vi "Spanning.vi"(6 "Numeric":i32, 8 "error in":errorcluster, 9 "TDMS File Ref":path, 10 "Log Start Time":timestamp, 11 "File Log Specification":T1={"Directory"=path "", "Groups"=[], "Buffer Size"=0, "Properties"=[], "Pretrigger"=FALSE, "Name"="", "Timestamp"=FALSE, "Error"=0, "Auto Open"=FALSE, "File Node Ref"=18446744073709551615, "Archive"=FALSE, "Archive Directory"=path "", "Span by Time"=FALSE, "Maximum Log Time"=86400, "Span by Size"=FALSE, "Maximum File Size"=100000} {"File Node Ref" format="%.0x"}) -> (0 "error out":errorcluster, 3 "Span File":bool)   [LabVIEW 2018, in "Embedded Data Logger Engine.lvlib"]
uses:
  Embedded Data Logger Engine.lvlib
  File Logging Specification.ctl
  Group Logging Specification.ctl
  Group Buffer Data.ctl
  Property Specification.ctl
  <vilib>/NI Veristand/Custom Device API/Custom Device Item Ref.ctl
  <vilib>/NI Veristand/Custom Device API/Custom Device API.lvlib
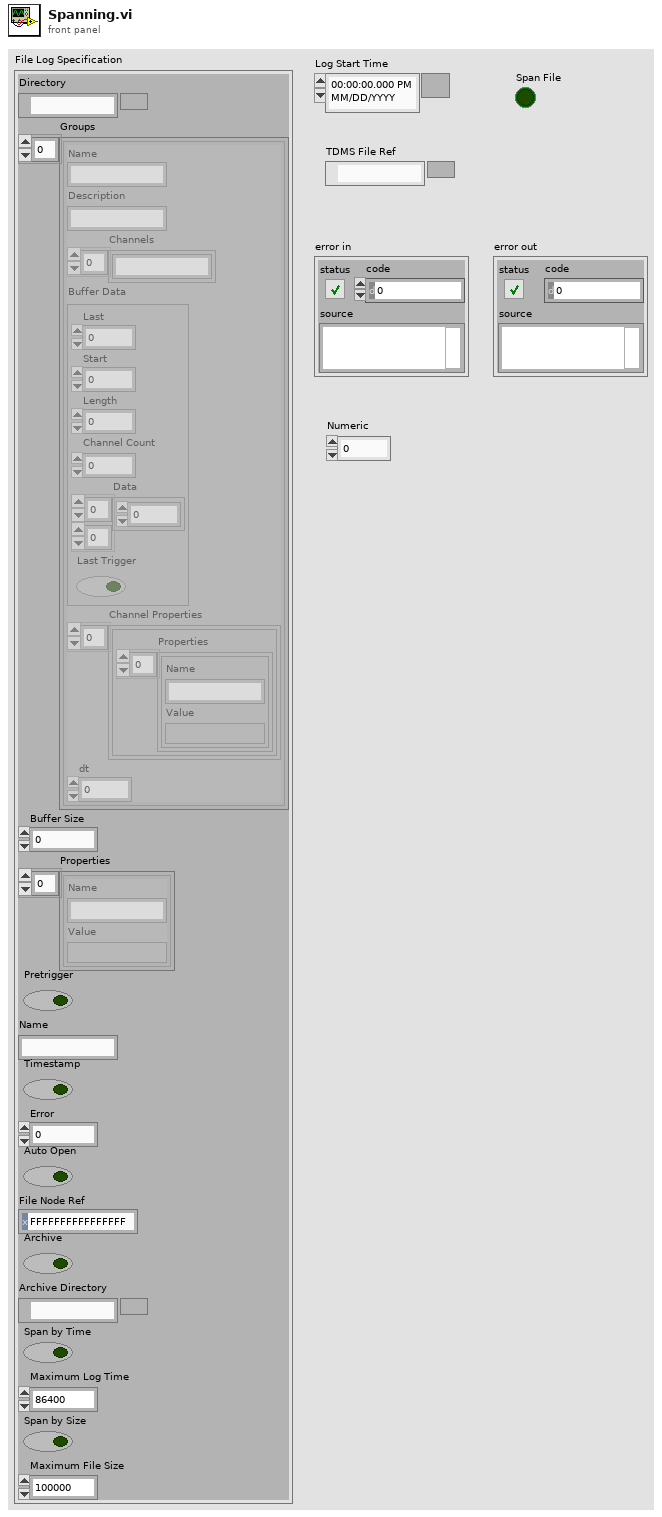
[diagram p1: front panel]
types:
  T1 = typedef "Embedded Data Logger Engine.lvlib/File Logging Specification.ctl" = cluster{"Directory":path, "Groups":T2[], "Buffer Size":i32, "Properties":T4[], "Pretrigger":bool, "Name":string, "Timestamp":bool, "Error":i32, "Auto Open":bool, "File Node Ref":T5, "Archive":bool, "Archive Directory":path, "Span by Time":bool, "Maximum Log Time":u32, "Span by Size":bool, "Maximum File Size":u32}
  T2 = typedef "Embedded Data Logger Engine.lvlib/Group Logging Specification.ctl" = cluster{"Name":string, "Description":string, "Channels":string[], "Buffer Data":T3, "Channel Properties":cluster{"Properties":T4[]}[], "dt":dbl}
  T3 = typedef "Embedded Data Logger Engine.lvlib/Group Buffer Data.ctl" = cluster{"Last":i32, "Start":i32, "Length":i32, "Channel Count":i32, "Data":dbl[][], "Last Trigger":bool}
  T4 = typedef "Embedded Data Logger Engine.lvlib/Property Specification.ctl" = cluster{"Name":string, "Value":variant}
  T5 = typedef "Custom Device API.lvlib/Custom Device Item Ref.ctl" = u64
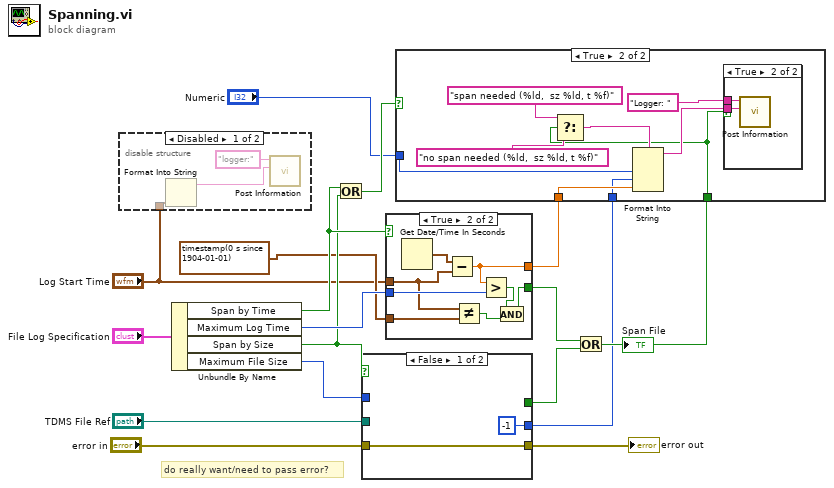
[diagram p0: block diagram]
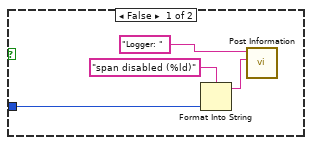
[diagram p3: hidden frame]
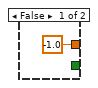
[diagram p5: hidden frame]
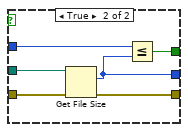
[diagram p6: hidden frame]
diagram:
  # "do really want/need to pass error?"
  n1 = disable-structure shown="Disabled" {
    disable-tunnel: "Log Start Time" -> [w19 _]
    frame Disabled {
      n2 = Format Into String(w19) -> (resulting string=w18:string)  [unwired: 3 in, 1 out]
      n3 = call "Post Information.vi"("Message"=w18, "Custom Device Name"="logger:") -> ()  [unwired: 9 in, 1 out]
    }
    frame Enabled {
    }
  }
  n4 = Unbundle By Name("File Log Specification") -> ("Span by Time"=w9:bool, "Maximum Log Time"=w14:u32, "Span by Size"=w8:bool, "Maximum File Size"=w15:u32)
  n5 = Or(x=w9, y=w8) -> (x .or. y?=w7:bool)
  n6 = case shown="False" w8 {
    tunnel: "TDMS File Ref" -> [_ w28]
    tunnel: w15 -> [_ w27]
    tunnel: [_ w26] -> w12
    tunnel: "error in" -> [w22 w25]
    tunnel: [w22 w24] -> w10
    tunnel: [i64 -1 ("size (in bytes)") w23] -> w3
    frame False {
    }
    frame True {
      n7 = Get File Size(file=w28, error in=w25) -> (size (in bytes)=w23:i64, 0:w24:errorcluster)  [unwired: 1 out]
      n8 = Less Or Equal?(x=w27, y=w23) -> (x <= y?=w26:bool)
    }
  }
  "error out" <- w10
  n9 = case shown="True" w9 {
    tunnel: "Log Start Time" -> [_ w32]
    tunnel: w14 -> [_ w36]
    tunnel: [_ w30] -> w13
    tunnel: [-1.0 w35] -> w4
    tunnel: timestamp(0 s since 1904-01-01) ("Log Start Time") -> [_ w31]
    frame False {
    }
    frame True {
      n10 = Get Date/Time In Seconds() -> (seconds since 1Jan1904=w37:timestamp)
      n11 = Subtract(x=w37, y=w32) -> (x-y=w35:dbl)
      n12 = Not Equal?(x=w32, y=w31) -> (x != y?=w33:bool)
      n13 = Greater?(x=w35, y=w36) -> (0:w34:bool)
      n14 = And(x=w34, y=w33) -> (x .and. y?=w30:bool)
    }
  }
  n15 = Or(x=w13, y=w12) -> (x .or. y?=w6:bool)
  "Span File" <- w6
  n16 = case shown="True" w7 {
    tunnel: w6 -> [_ w42]
    tunnel: "Numeric" -> [w39 w46]
    tunnel: w4 -> [_ w44]
    tunnel: w3 -> [_ w43]
    frame False {
      n17 = Format Into String(format string="span disabled (%ld)" ("Message"), w39) -> (resulting string=w38:string)  [unwired: 2 in, 1 out]
      n18 = call "Post Information.vi"("Message"=w38, "Custom Device Name"="Logger: ") -> ()  [unwired: 9 in, 1 out]
    }
    frame True {
      n19 = Select(t="span needed (%ld,  sz %ld, t %f)" ("Custom Device Name"), s=w42, f="no span needed (%ld,  sz %ld, t %f)" ("Custom Device Name")) -> (s? t:f=w47:string)
      n20 = Format Into String(format string=w47, w46, w43, w44) -> (resulting string=w45:string)  [unwired: 2 in, 1 out]
      n21 = case shown="True" w42 {
        tunnel: "Logger: " ("Custom Device Name") -> [_ w52]
        tunnel: w45 -> [_ w51]
        frame False {
        }
        frame True {
          n22 = call "Post Information.vi"("Message"=w51, "Custom Device Name"=w52) -> ()  [unwired: 9 in, 1 out]
        }
      }
    }
  }
